vi "Btolerance.vi"(0 "index":ext[](array[numeric]), 1 "tolerance (B)":dbl=0.001, 5 "time":ext[](array[numeric]), 7 "dB/dt":ext[](array[numeric]), 9 "B":ext[](array[numeric]), 11 "data":dbl[](array[numeric])) -> (4 "index 2":ext[](array[numeric]), 6 "time 2":ext[](array[numeric]), 8 "dB/dt 2":ext[](array[numeric]), 10 "B 2":ext[](array[numeric]), 15 "data 2":dbl[](array[numeric]))   [LabVIEW 2015]
uses:
  <vilib>/Analysis/baseanly.llb/Mean (DBL).vi
  <vilib>/Analysis/NI_AALBase.lvlib
panel:
  in  "Array":dbl[](array[numeric])
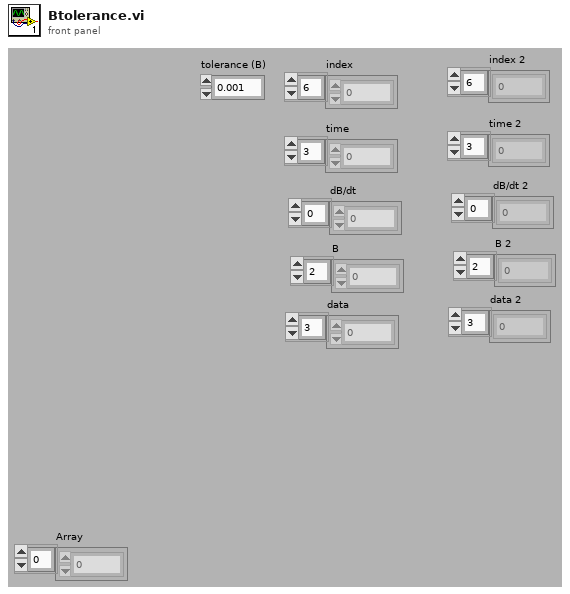
[diagram p1: front panel]
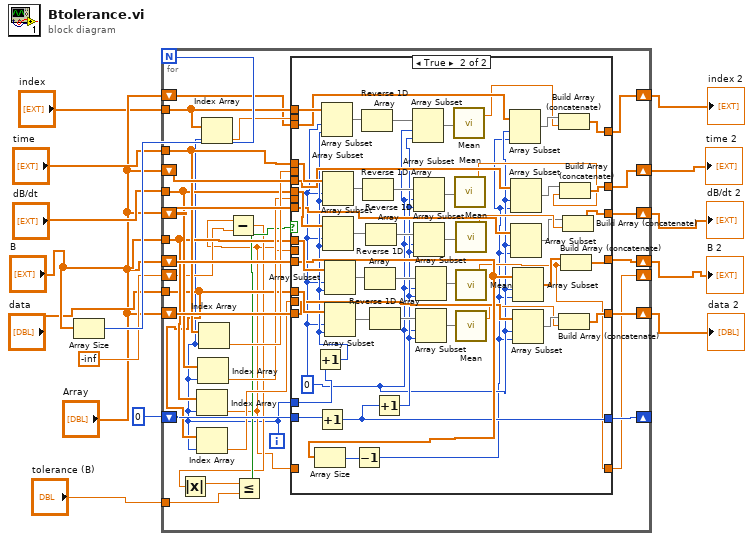
[diagram p0: block diagram]
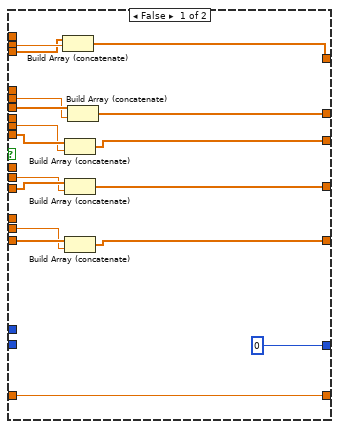
[diagram p2: hidden frame]
diagram:
  n1 = Array Size(array="B") -> (size(s)=w15:i32)
  n2 = for {
    N: w15 -> [_]
    shift-right: [w40] -> w7
    shift-left: "Array" -> [w44]
    shift-right: [w39] -> w6
    shift-left: "Array" -> [w43]
    shift-right: [w38] -> w5
    shift-left: "Array" -> [w42]
    shift-right: [w37] -> w4
    shift-left: "Array" -> [w41]
    shift-right: [w22] -> _
    shift-left: -inf -> [w27]
    shift-right: [w35] -> _
    shift-left: 0 -> [w36]
    tunnel: "time" -> [w34]
    tunnel: "dB/dt" -> [w32]
    tunnel: "B" -> [w30]
    tunnel: "data" -> [w29]
    tunnel: "tolerance (B)" -> [w25]
    shift-right: [w16] -> w1
    shift-left: "Array" -> [w17]
    tunnel: "index" -> [w20]
    i -> [w19]
    n3 = Index Array(array=w30, index=w19) -> (element=w21:ext)
    n4 = Index Array(array=w29, index=w19) -> (element=w28:dbl)
    n5 = Index Array(array=w32, index=w19) -> (element=w31:ext)
    n6 = Index Array(array=w34, index=w19) -> (element=w33:ext)
    n7 = Index Array(array=w20, index=w19) -> (element=w18:ext)
    n8 = Subtract(x=w21, y=w27) -> (x-y=w23:ext)
    n9 = Absolute Value(x=w23) -> (abs(x)=w26:ext)
    n10 = Less Or Equal?(x=w26, y=w25) -> (x <= y?=w24:bool)
    n11 = case shown="True" w24 {
      tunnel: w44 -> [w61 w91]
      tunnel: w43 -> [w60 w90]
      tunnel: w42 -> [w59 w89]
      tunnel: w41 -> [w58 w88]
      tunnel: [w57 w80] -> w40
      tunnel: w33 -> [w56 _]
      tunnel: w31 -> [w55 _]
      tunnel: w21 -> [w54 _]
      tunnel: w28 -> [w53 _]
      tunnel: [w52 w81] -> w39
      tunnel: [w51 w82] -> w38
      tunnel: [w50 w83] -> w37
      tunnel: w36 -> [_ w109]
      tunnel: [0 w77] -> w35
      tunnel: w34 -> [_ w107]
      tunnel: w32 -> [_ w106]
      tunnel: w30 -> [_ w105]
      tunnel: w29 -> [_ w104]
      tunnel: w19 -> [_ w76]
      tunnel: w21 -> [w48 _]
      tunnel: [w48 w75] -> w22
      tunnel: w20 -> [_ w69]
      tunnel: w18 -> [w47 _]
      tunnel: w17 -> [w46 w68]
      tunnel: [w45 w64] -> w16
      frame False {
        n12 = Build Array (concatenate)(w46, w47) -> (w45:ext[])
        n13 = Build Array (concatenate)(w60, w55) -> (w52:ext[])
        n14 = Build Array (concatenate)(w59, w54) -> (w51:ext[])
        n15 = Build Array (concatenate)(w58, w53) -> (w50:dbl[])
        n16 = Build Array (concatenate)(w61, w56) -> (w57:ext[])
      }
      frame True {
        w63 = 0
        n17 = Increment(x=w76) -> (x+1=w67:i32)
        n18 = Array Size(array=w89) -> (size(s)=w92:i32)
        n19 = Increment(x=w109) -> (x+1=w77:i32)
        n20 = Array Subset(array=w69, index=w63, length=w67) -> (w73:ext[])
        n21 = Array Subset(array=w107, index=w63, length=w67) -> (w108:ext[])
        n22 = Array Subset(array=w106, index=w63, length=w67) -> (w103:ext[])
        n23 = Array Subset(array=w105, index=w63, length=w67) -> (w102:ext[])
        n24 = Array Subset(array=w104, index=w63, length=w67) -> (w101:dbl[])
        n25 = Decrement(x=w92) -> (x-1=w62:i32)
        n26 = Reverse 1D Array(array=w73) -> (reversed array=w72:ext[])
        n27 = Reverse 1D Array(array=w108) -> (reversed array=w100:ext[])
        n28 = Reverse 1D Array(array=w102) -> (reversed array=w98:ext[])
        n29 = Reverse 1D Array(array=w103) -> (reversed array=w99:ext[])
        n30 = Reverse 1D Array(array=w101) -> (reversed array=w97:dbl[])
        n31 = Increment(x=w77) -> (x+1=w66:i32)
        n32 = Array Subset(array=w72, index=w63, length=w66) -> (w71:ext[])
        n33 = Array Subset(array=w100, index=w63, length=w66) -> (w96:ext[])
        n34 = Array Subset(array=w99, index=w63, length=w66) -> (w95:ext[])
        n35 = Array Subset(array=w98, index=w63, length=w66) -> (w94:ext[])
        n36 = Array Subset(array=w97, index=w63, length=w66) -> (w93:dbl[])
        n37 = call-poly <vilib>:"Mean.vi"("X"=w71) -> ("mean"=w65:dbl)  [unwired: 1 out]
        n38 = call-poly <vilib>:"Mean.vi"("X"=w96) -> ("mean"=w74:dbl)  [unwired: 1 out]
        n39 = call-poly <vilib>:"Mean.vi"("X"=w95) -> ("mean"=w84:dbl)  [unwired: 1 out]
        n40 = call-poly <vilib>:"Mean.vi"("X"=w94) -> ("mean"=w75:dbl)  [unwired: 1 out]
        n41 = call-poly <vilib>:"Mean.vi"("X"=w93) -> ("mean"=w85:dbl)  [unwired: 1 out]
        n42 = Array Subset(array=w68, index=w63, length=w62) -> (w70:ext[])
        n43 = Array Subset(array=w91, index=w63, length=w62) -> (w87:ext[])
        n44 = Array Subset(array=w90, index=w63, length=w62) -> (w79:ext[])
        n45 = Array Subset(array=w89, index=w63, length=w62) -> (w78:ext[])
        n46 = Array Subset(array=w88, index=w63, length=w62) -> (w86:dbl[])
        n47 = Build Array (concatenate)(w70, w65) -> (w64:ext[])
        n48 = Build Array (concatenate)(w86, w85) -> (w83:dbl[])
        n49 = Build Array (concatenate)(w87, w74) -> (w80:ext[])
        n50 = Build Array (concatenate)(w78, w75) -> (w82:ext[])
        n51 = Build Array (concatenate)(w79, w84) -> (w81:ext[])
      }
    }
  }
  "time 2" <- w7
  "dB/dt 2" <- w6
  "B 2" <- w5
  "data 2" <- w4
  "index 2" <- w1
